vi "setAO.vi"(8 "错误输入（无错误）":errorcluster, 9 "value":dbl, 10 "channel":i32) -> (0 "错误输出":errorcluster)   [LabVIEW 2013]
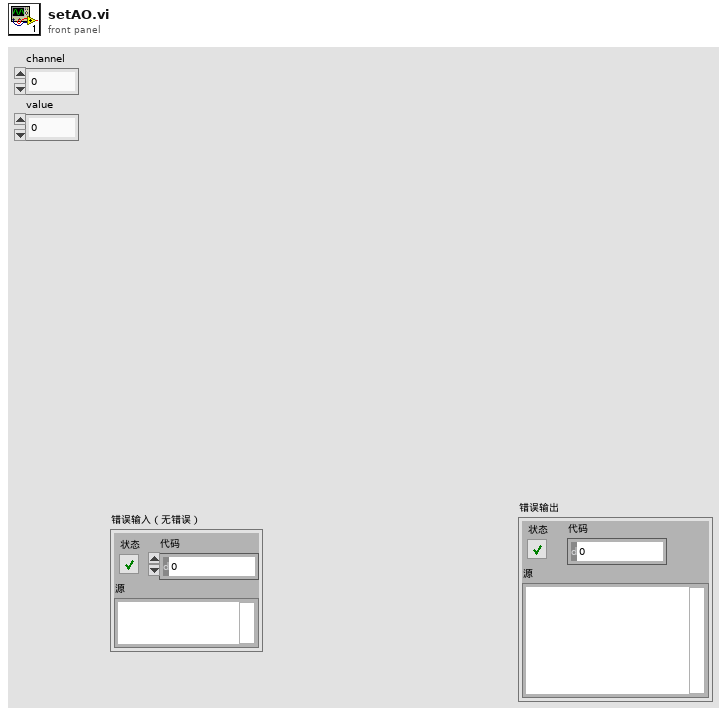
[diagram p1: front panel]
types:
  T1 = cluster{"cmd":string, "channel":i32, "value":dbl, "on/off":bool, "return value":refnum<vi>}
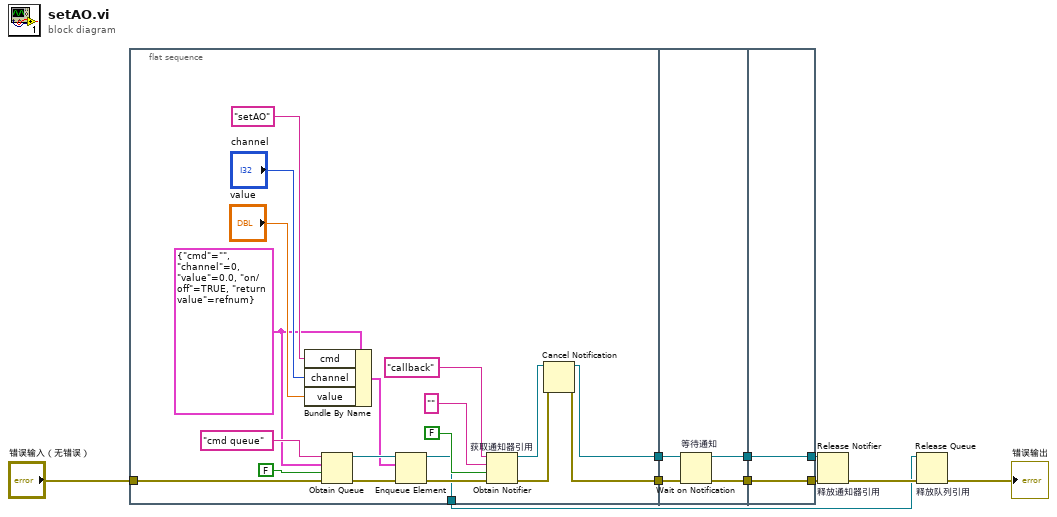
[diagram p0: block diagram]
diagram:
  n1 = flat-sequence {
    tunnel: [w13] -> w10
    tunnel: [w11] -> w9
    tunnel: "错误输入（无错误）" -> [w21]
    tunnel: [w15] -> w2
    tunnel: w10 -> [w33]
    tunnel: w9 -> [w32]
    tunnel: [w31] -> w8
    tunnel: [w30] -> w6
    tunnel: w8 -> [w35]
    tunnel: [w35] -> w7
    tunnel: w6 -> [w34]
    tunnel: [w34] -> w5
    frame #0 {
      w18 = T1 {"cmd"="", "channel"=0, "value"=0.0, "on/off"=TRUE, "return value"=refnum}
      n2 = Bundle By Name(cluster=w18, "cmd"="setAO", "channel"="channel", "value"="value") -> (w17:T1)
      n3 = Obtain Queue(name (unnamed)="cmd queue" ("名称（未命名）"), element data type=w18, create if not found? (T)=FALSE ("如未找到是否创建？(T)"), error in (no error)=w21) -> (queue out=w19:refnum<queue>, error out=w20:errorcluster)  [unwired: 1 in, 1 out]
      n4 = Enqueue Element(queue=w19, element=w17, error in (no error)=w20) -> (queue out=w15:refnum<queue>, error out=w16:errorcluster)  [unwired: 1 in, 1 out]
      n5 = Obtain Notifier "获取通知器引用"(name (unnamed)="callback" ("名称（未命名）"), notification data type="", create if not found? (T)=FALSE ("如未找到是否创建？(T)"), error in (no error)=w16) -> (notifier out=w14:refnum<notifier>, error out=w12:errorcluster)  [unwired: 1 out]
      n6 = Cancel Notification(0:w14, 3:w12) -> (8:w13:refnum<notifier>, 11:w11:errorcluster)  [unwired: 1 out]
    }
    frame #1 {
      n7 = Wait on Notification "等待通知"(notifier=w33, error in (no error)=w32) -> (notifier out=w31:refnum<notifier>, error out=w30:errorcluster)  [unwired: 2 in, 2 out]
    }
    frame #2 {
    }
  }
  n8 = Release Notifier "释放通知器引用"(notifier=w7, error in (no error)=w5) -> (error out=w3:errorcluster)  [unwired: 1 in, 2 out]
  n9 = Release Queue "释放队列引用"(queue=w2, error in (no error)=w3) -> (error out=→"错误输出":errorcluster)  [unwired: 1 in, 2 out]
